vi "get_configuration.vi"(8 "error in (no error)":errorcluster, 11 "ErrorController in":refnum<class "ErrorController.lvclass">) -> (0 "error out":errorcluster, 2 "target configuration file out":path, 3 "ErrorController out":refnum<class "ErrorController.lvclass">)   [LabVIEW 2010, in "ErrorController.lvclass"]
uses:
  ErrorController.lvclass
  ErrorController.lvclass/ErrorController.ctl
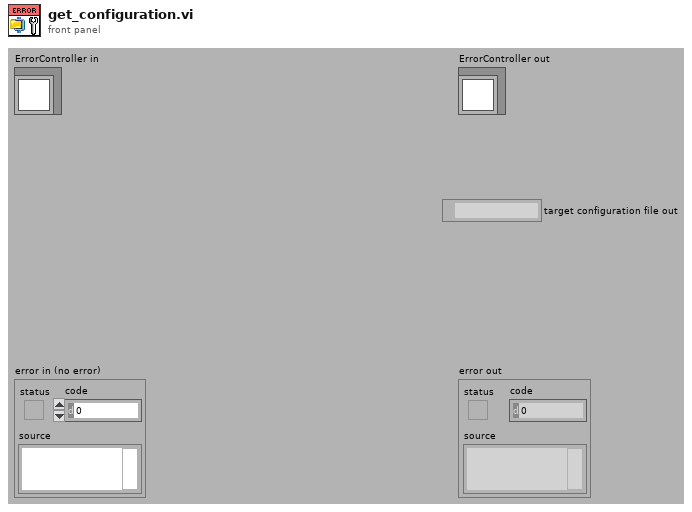
[diagram p1: front panel]
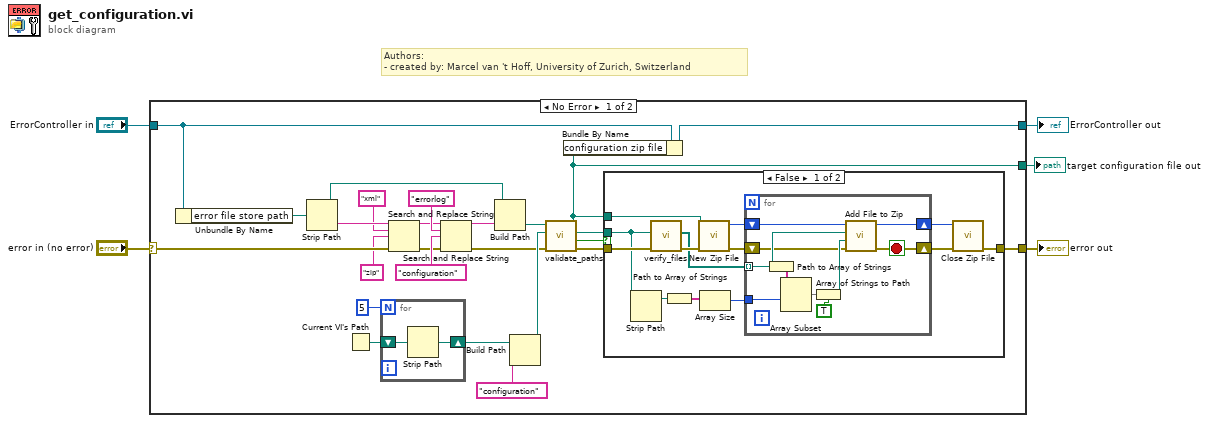
[diagram p0: block diagram]
diagram:
  # "Authors: \n- created by: Marcel van 't Hoff, University of Zurich, Switzerland"
  n1 = case shown="No Error" "error in (no error)" {
    selector: "error in (no error)" -> [w14 w58]
    tunnel: [w30 w58] -> w4
    tunnel: [w17 w57] -> w2
    tunnel: "ErrorController in" -> [w18 w57]
    tunnel: [w16 _] -> w1
    frame No Error {
      n2 = Unbundle By Name(w18) -> ("error file store path"=w19:path)
      n3 = Strip Path(path=w19) -> (stripped path=w25:path, name=w15:string)
      n4 = Current VI's Path() -> (path=w29:path)
      n5 = for {
        N: 5 -> [_]
        shift-right: [w55] -> w27
        shift-left: w29 -> [w56]
        n6 = Strip Path(path=w56) -> (stripped path=w55:path)  [unwired: 1 out]
      }
      n7 = Search and Replace String(input string=w15, search string="xml", replace string="zip" ("replace string (\"\")"), error in=w14) -> (result string=w8:string, error out=w9:errorcluster)  [unwired: 4 in, 2 out]
      n8 = Search and Replace String(input string=w8, search string="errorlog", replace string="configuration" ("replace string (\"\")"), error in=w9) -> (result string=w6:string, error out=w7:errorcluster)  [unwired: 4 in, 2 out]
      n9 = Build Path(base path=w25, name or relative path=w6) -> (appended path=w21:path)
      n10 = Build Path(base path=w27, name or relative path="configuration") -> (appended path=w20:path)
      n11 = call "validate_paths.vi"("error in (no error)"=w7, "File or Directory input"=w20, "Target zip file input"=w21) -> ("error out"=w23:errorcluster, "Invalid Path?"=w22:bool, "File or Directory selected"=w24:path, "Target zip file selected"=w16:path)  [unwired: 5 in]
      n12 = Bundle By Name(cluster=w18, "configuration zip file"=w16) -> (w17:refnum<class "ErrorController.lvclass">)
      n13 = case shown="False" w22 {
        tunnel: w24 -> [w38 _]
        tunnel: w23 -> [w43 w54]
        tunnel: w16 -> [w41 _]
        tunnel: [w31 w54] -> w30
        frame False {
          n14 = Strip Path(path=w38) -> (stripped path=w39:path)  [unwired: 1 out]
          n15 = call "verify_files.vi"("error in (no error)"=w43, "File or Directory"=w38) -> ("error out"=w42:errorcluster, "Array"=w37:path[])  [unwired: 8 in]
          n16 = Path to Array of Strings(0:w39) -> (2:w40:string[])  [unwired: 1 out]
          n17 = call <vilib>:"New Zip File.vi"("error in (no error)"=w42, "target"=w41) -> ("error out"=w34:errorcluster, "zip file out"=w36:i64)  [unwired: 3 in, 1 out]
          n18 = Array Size(array=w40) -> (size(s)=w35:i32)
          n19 = for {
            tunnel: w37 -> [w49] mode=indexing
            tunnel: w35 -> [w50]
            shift-right: [w46] -> w33
            shift-left: w34 -> [w47]
            shift-right: [w44] -> w32
            shift-left: w36 -> [w45]
            stop <- w46 stop-if-true
            n20 = Path to Array of Strings(0:w49) -> (2:w51:string[])  [unwired: 1 out]
            n21 = Array Subset(array=w51, index=w50) -> (w52:string[])  [unwired: 1 in]
            n22 = Array of Strings to Path(0:w52, 1:TRUE ("relative")) -> (2:w48:path)
            n23 = call <vilib>:"Add File to Zip.vi"("error in (no error)"=w47, "destination path in zip"=w48, "source file path"=w49, "zip file in"=w45) -> ("error out"=w46:errorcluster, "zip file out"=w44:i64)  [unwired: 6 in]
          }
          n24 = call <vilib>:"Close Zip File.vi"("error in (no error)"=w33, "zip file in"=w32) -> ("error out"=w31:errorcluster)  [unwired: 5 in]
        }
        frame True {
        }
      }
    }
    frame Error {
    }
  }
  "error out" <- w4
  "ErrorController out" <- w2
  "target configuration file out" <- w1
